vi "Software licence Manager Inputs.vi"(8 "error in (no error)":errorcluster) -> (0 "error out":errorcluster, 3 "Software Licence Manager Inputs Out":T1)   [LabVIEW 2015]
uses:
  <vilib>/Utility/config.llb/Read Key (String).vi
  <vilib>/Utility/config.llb/NI_LVConfig.lvlib
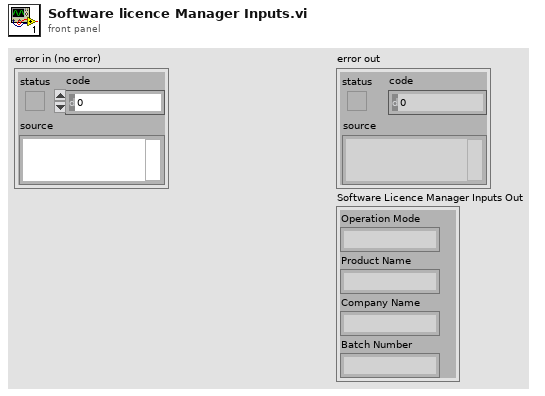
[diagram p1: front panel]
types:
  T1 = cluster{"Operation Mode":string, "Product Name":string, "Company Name":string, "Batch Number":string}
  T2 = typedef "NI_LVConfig.lvlib/Config Data RefNum.ctl" = refnum<k1>
  T3 = cluster{"value":string, "value":string, "value":string, "value":string}
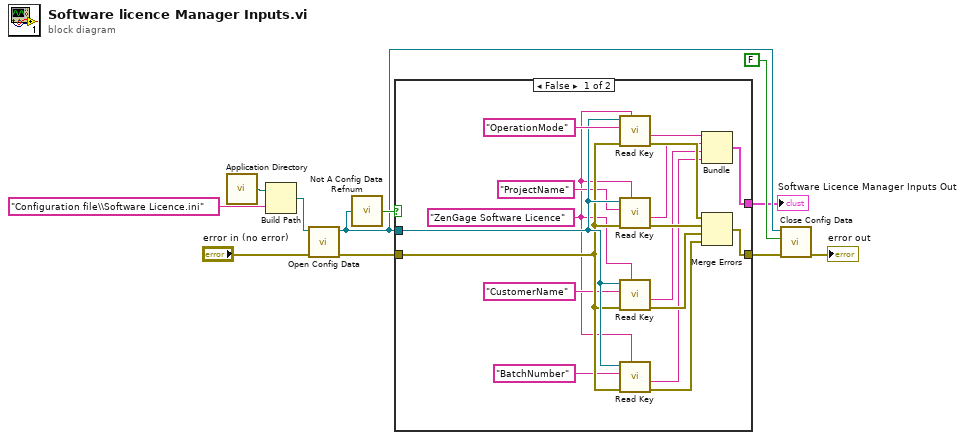
[diagram p0: block diagram]
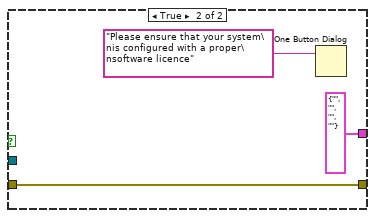
[diagram p2: hidden frame]
diagram:
  n1 = call <vilib>:"Application Directory.vi"() -> ("Application Directory"=w11:path)
  n2 = Build Path(base path=w11, name or relative path="Configuration file\\Software Licence.ini") -> (appended path=w9:path)
  n3 = call <vilib>:"Open Config Data.vi"("error in (no error)"="error in (no error)", "configuration file path"=w9) -> ("error out"=w6:errorcluster, "refnum"=w4:T2)  [unwired: 7 in, 1 out]
  n4 = call <vilib>:"Not A Config Data Refnum.vi"("refnum"=w4) -> ("not a config data refnum"=w7:bool)
  n5 = case shown="False" w7 {
    tunnel: w4 -> [w27 _]
    tunnel: w6 -> [w26 w30]
    tunnel: [w18 w30] -> w5
    tunnel: [w13 T3 {"value"="", "value"="", "value"="", "value"=""}] -> w1
    frame False {
      w12 = "ZenGage Software Licence" ("section")
      n6 = call-poly <vilib>:"Read Key.vi"("section"=w12, "error in (no error)"=w26, "key"="OperationMode", "refnum"=w27) -> ("error out"=w22:errorcluster, "value"=w17:string)  [unwired: 4 in, 2 out]
      n7 = call-poly <vilib>:"Read Key.vi"("section"=w12, "error in (no error)"=w26, "key"="ProjectName", "refnum"=w27) -> ("error out"=w21:errorcluster, "value"=w16:string)  [unwired: 4 in, 2 out]
      n8 = call-poly <vilib>:"Read Key.vi"("section"=w12, "error in (no error)"=w26, "key"="CustomerName", "refnum"=w27) -> ("error out"=w20:errorcluster, "value"=w15:string)  [unwired: 4 in, 2 out]
      n9 = call-poly <vilib>:"Read Key.vi"("section"=w12, "error in (no error)"=w26, "key"="BatchNumber", "refnum"=w27) -> ("error out"=w19:errorcluster, "value"=w14:string)  [unwired: 4 in, 2 out]
      n10 = Bundle("value"=w17, "value"=w16, "value"=w15, "value"=w14) -> (w13:T3)  [unwired: 1 in]
      n11 = Merge Errors(w22, w21, w20, w19) -> (w18:errorcluster)
    }
    frame True {
      n12 = One Button Dialog(message="Please ensure that your system\nis configured with a proper\nsoftware licence") -> ()  [unwired: 1 in, 1 out]
    }
  }
  "Software Licence Manager Inputs Out" <- w1
  n13 = call <vilib>:"Close Config Data.vi"("error in (no error)"=w5, "write file if changed (T)"=FALSE, "refnum"=w4) -> ("error out"=→"error out":errorcluster)  [unwired: 7 in, 1 out]
